vi "Test AWG.vi"() -> ()   [LabVIEW 2024]
uses:
  Ramps.ctl
panel:
  in  "AWG test parameter":T1={"Amp"=1.0, "Delay time 10us"=1000, "Ramp1 time 10us"=2000, "Ramp2 time 10us"=10, "Ramp3 time 10us"=500, "End time 10us"=10}
  in  "Update":bool
  in  "stop":bool
  in  "error in (no error)":errorcluster
  out "DAQ_AI_Reader endpoint":refnum<k21>="DAQ_AI_Reader"
  out "DAQ_CMD_Writer endpoint":refnum<k21>="DAQ_CMD_Writer"
  in  "cRIO IP":string="//172.22.11.2"
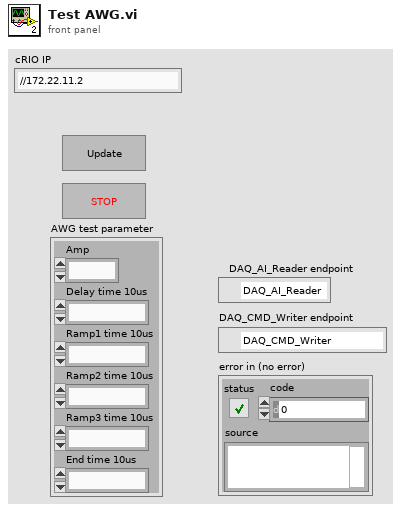
[diagram p1: front panel]
types:
  T1 = typedef "Ramps.ctl" = cluster{"Amp":fxp<+/-,20,5>, "Delay time 10us":i32, "Ramp1 time 10us":i32, "Ramp2 time 10us":i32, "Ramp3 time 10us":i32, "End time 10us":i32}
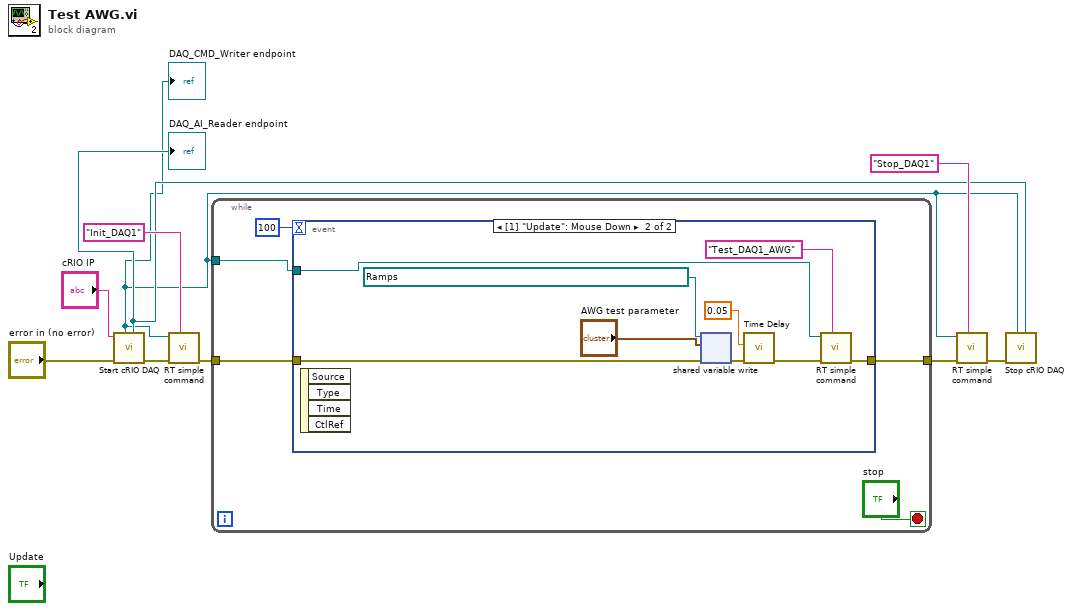
[diagram p0: block diagram]
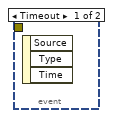
[diagram p2: hidden frame]
diagram:
  n1 = call "Start cRIO DAQ.vi"("error in (no error)"="error in (no error)", "cRIO IP"="cRIO IP") -> ("error out"=w3:errorcluster, "DAQ_AI_Reader endpoint"=w6:refnum<k21>, "DAQ_CMD_Writer endpoint"=w1:refnum<k21>)  [unwired: 7 in]
  "DAQ_CMD_Writer endpoint" <- w1
  "DAQ_AI_Reader endpoint" <- w6
  n2 = call "RT simple command.vi"("Command"="Init_DAQ1", "error in (no error)"=w3, "DAQ_CMD_Writer endpoint"=w1) -> ("error out"=w2:errorcluster)  [unwired: 7 in, 1 out]
  n3 = while {
    tunnel: [w13] -> w5
    tunnel: w2 -> [w12]
    tunnel: w1 -> [w11]
    stop <- "stop" stop-if-true
    n4 = event shown="[1] \"Update\": Mouse Down" {
      selector: _ -> [_ _]
      dyn-events: _ -> [_ _]
      timeout: 100 -> [_ _]
      tunnel: [_ w23] -> w13
      tunnel: w12 -> [_ w20]
      tunnel: w11 -> [_ w22]
      event Timeout {
        n5 = event-data() -> ()  [unwired: 1 in, 3 out]
      }
      event "Update": Mouse Down {
        n6 = event-data() -> ()  [unwired: 1 in, 4 out]
        n7 = shared-variable-write(refnum<k21> "ni.var.psp://172.22.11.2/network varibles/AWG test ramp" ("shared variable refnum in"), w20, "AWG test parameter") -> (w19:errorcluster)  [unwired: 1 out]
        n8 = call "Time Delay"("error in (no error)"=w19, "Delay Time (s)"=0.05) -> ("error out"=w18:errorcluster)  [unwired: 9 in]
        n9 = call "RT simple command.vi"("Command"="Test_DAQ1_AWG", "error in (no error)"=w18, "DAQ_CMD_Writer endpoint"=w22) -> ("error out"=w23:errorcluster)  [unwired: 7 in, 1 out]
      }
    }
  }
  n10 = call "RT simple command.vi"("Command"="Stop_DAQ1", "error in (no error)"=w5, "DAQ_CMD_Writer endpoint"=w1) -> ("error out"=w8:errorcluster)  [unwired: 7 in, 1 out]
  n11 = call "Stop cRIO DAQ.vi"("DAQ_AI_Reader endpoint"=w6, "DAQ_CMD_Writer endpoint"=w1, "error in (no error)"=w8) -> ()  [unwired: 8 in, 1 out]
